vi "XML_EEG_writeHeader.vi"(8 "error in (no error)":errorcluster, 10 "XML_Header":T1, 11 "XML_EEG_File in":refnum<class "XML_EEG_File.lvclass">) -> (0 "error out":errorcluster, 2 "DOM document out":refnum<k20>, 3 "XML_EEG_File out":refnum<class "XML_EEG_File.lvclass">)   [LabVIEW 2016, in "XML_EEG_File_Parser.lvlib" / "XML_EEG_File.lvclass"]
uses:
  XML_EEG_File.lvclass
  XML_EEG_Header.ctl
  XML_EEG_File.lvclass/XML_EEG_File.ctl
  <vilib>/xml/NI_XML.lvlib
  <resource>/objmgr/DOMUserDefRef.rc
  XML_EEG_File_Parser.lvlib
panel:
  # "This VI is a part of BCI Design library, http://www.ru-bci.org \nCopyright © 2020, Sotnikov Peter, All rights reserved. License: CC BY-NC 4.0"
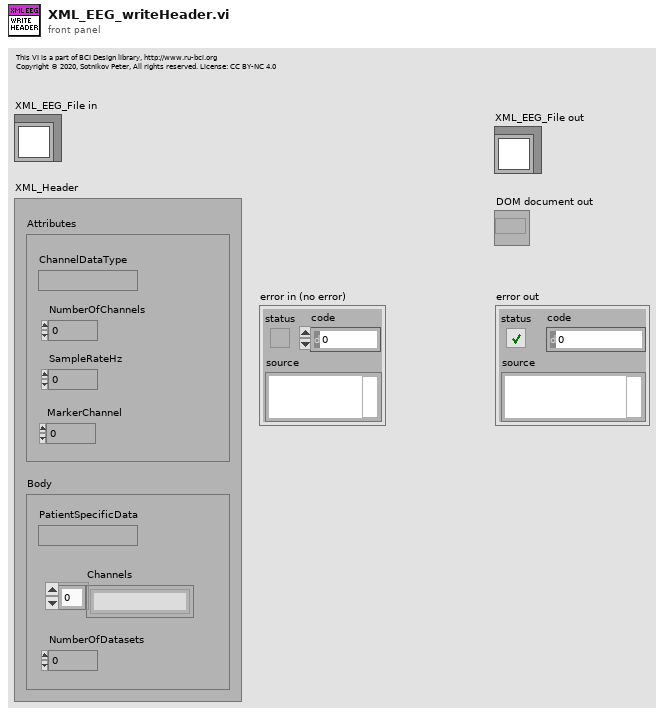
[diagram p1: front panel]
types:
  T1 = typedef "XML_EEG_File_Parser.lvlib/XML_EEG_Header.ctl" = cluster{"Attributes":cluster{"ChannelDataType":string, "NumberOfChannels":i32, "SampleRateHz":dbl, "MarkerChannel":i32}, "Body":cluster{"PatientSpecificData":string, "NumberOfDatasets":i32, "Channels":string[]}}
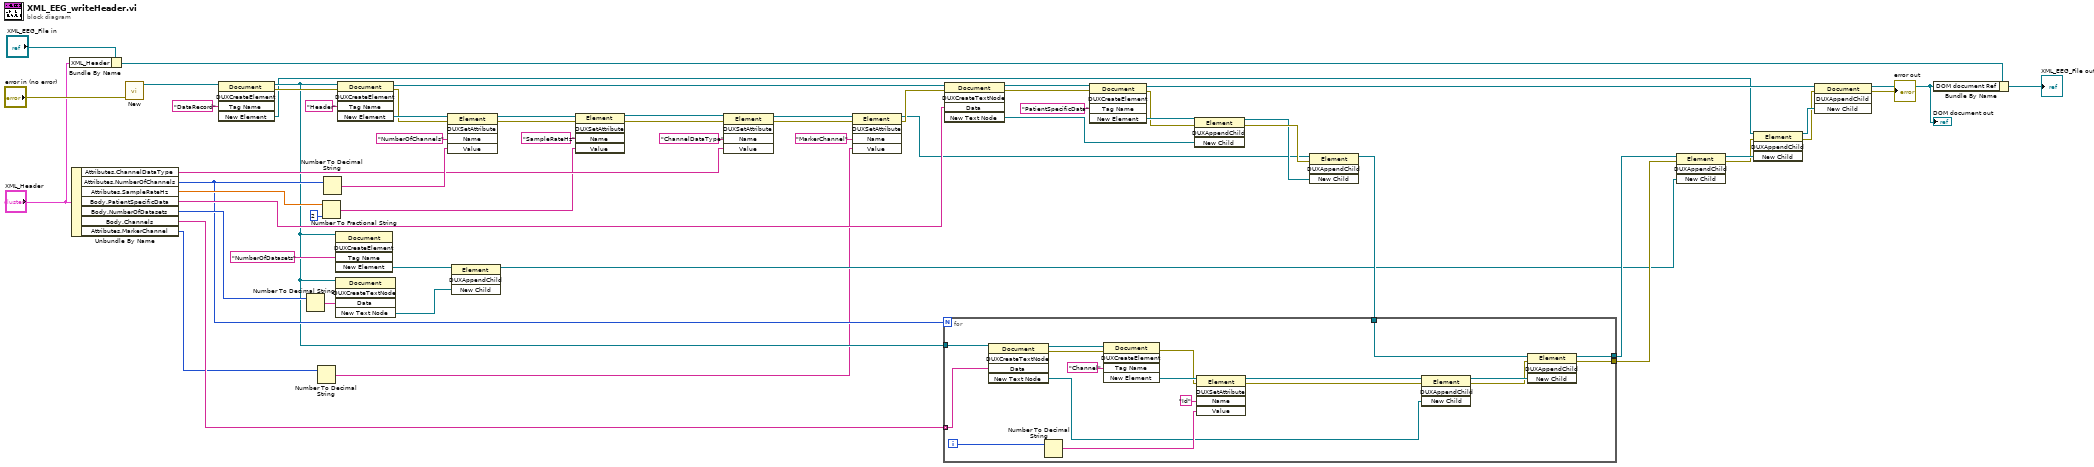
[diagram p0: block diagram]
diagram:
  n1 = Bundle By Name(cluster="XML_EEG_File in", "XML_Header"="XML_Header") -> (w3:refnum<class "XML_EEG_File.lvclass">)
  n2 = Unbundle By Name("XML_Header") -> ("Attributes.ChannelDataType"=w46:string, "Attributes.NumberOfChannels"=w26:i32, "Attributes.SampleRateHz"=w45:dbl, "Body.PatientSpecificData"=w41:string, "Body.NumberOfDatasets"=w30:i32, "Body.Channels"=w27:string[], "Attributes.MarkerChannel"=w8:i32)
  n3 = call <vilib>:"New.vi"("error in (no error)"="error in (no error)") -> ("DOM document out"=w60:refnum<k20>)  [unwired: 7 in, 1 out]
  n4 = invoke class="Document" method="DUXCreateElement"(reference=w60, "Tag Name"="DataRecord") -> (reference out=w25:refnum<k20>, error out=w58:errorcluster, "New Element"=w17:refnum<k20>)  [unwired: 3 in, 2 out]
  n5 = Number To Decimal String(number=w30) -> (decimal integer string=w31:string)  [unwired: 1 in]
  n6 = Number To Decimal String(number=w8) -> (decimal integer string=w7:string)  [unwired: 1 in]
  n7 = Number To Fractional String(number=w45, precision (6)=i16 2) -> (F-format string=w43:string)  [unwired: 2 in]
  n8 = Number To Decimal String(number=w26) -> (decimal integer string=w47:string)  [unwired: 1 in]
  n9 = invoke class="Document" method="DUXCreateElement"(reference=w25, "Tag Name"="NumberOfDatasets") -> ("New Element"=w29:refnum<k20>)  [unwired: 3 in, 4 out]
  n10 = invoke class="Document" method="DUXCreateTextNode"(reference=w25, "Data"=w31) -> ("New Text Node"=w28:refnum<k20>)  [unwired: 3 in, 4 out]
  n11 = invoke class="Document" method="DUXCreateElement"(reference=w25, error in=w58, "Tag Name"="Header") -> (reference out=w42:refnum<k20>, error out=w54:errorcluster, "New Element"=w56:refnum<k20>)  [unwired: 2 in, 2 out]
  n12 = invoke class="Element" method="DUXSetAttribute"(reference=w56, error in=w54, "Name"="NumberOfChannels", "Value"=w47) -> (reference out=w53:refnum<k20>, error out=w52:errorcluster)  [unwired: 1 in, 3 out]
  n13 = invoke class="Element" method="DUXAppendChild"(reference=w29, "New Child"=w28) -> (reference out=w21:refnum<k20>)  [unwired: 2 in, 3 out]
  n14 = invoke class="Element" method="DUXSetAttribute"(reference=w53, error in=w52, "Name"="SampleRateHz", "Value"=w43) -> (reference out=w50:refnum<k20>, error out=w49:errorcluster)  [unwired: 1 in, 3 out]
  n15 = invoke class="Element" method="DUXSetAttribute"(reference=w50, error in=w49, "Name"="ChannelDataType", "Value"=w46) -> (reference out=w11:refnum<k20>, error out=w12:errorcluster)  [unwired: 1 in, 3 out]
  n16 = invoke class="Element" method="DUXSetAttribute"(reference=w11, error in=w12, "Name"="MarkerChannel", "Value"=w7) -> (reference out=w9:refnum<k20>, error out=w10:errorcluster)  [unwired: 1 in, 3 out]
  n17 = invoke class="Document" method="DUXCreateTextNode"(reference=w42, error in=w10, "Data"=w41) -> (reference out=w39:refnum<k20>, error out=w40:errorcluster, "New Text Node"=w35:refnum<k20>)  [unwired: 2 in, 2 out]
  n18 = invoke class="Document" method="DUXCreateElement"(reference=w39, error in=w40, "Tag Name"="PatientSpecificData") -> (reference out=w20:refnum<k20>, error out=w36:errorcluster, "New Element"=w37:refnum<k20>)  [unwired: 2 in, 2 out]
  n19 = invoke class="Element" method="DUXAppendChild"(reference=w37, error in=w36, "New Child"=w35) -> (reference out=w33:refnum<k20>, error out=w34:errorcluster)  [unwired: 1 in, 2 out]
  n20 = invoke class="Element" method="DUXAppendChild"(reference=w9, error in=w34, "New Child"=w33) -> (reference out=w24:refnum<k20>)  [unwired: 1 in, 3 out]
  n21 = for {
    N: w26 -> [_]
    tunnel: w27 -> [w63] mode=indexing
    tunnel: w25 -> [w72]
    tunnel: w24 -> [w66]
    tunnel: [w65] -> w23
    tunnel: [w64] -> w22
    i -> [w74]
    n22 = invoke class="Document" method="DUXCreateTextNode"(reference=w72, "Data"=w63) -> (reference out=w71:refnum<k20>, error out=w70:errorcluster, "New Text Node"=w69:refnum<k20>)  [unwired: 3 in, 2 out]
    n23 = Number To Decimal String(number=w74) -> (decimal integer string=w73:string)  [unwired: 1 in]
    n24 = invoke class="Document" method="DUXCreateElement"(reference=w71, error in=w70, "Tag Name"="Channel") -> (error out=w76:errorcluster, "New Element"=w77:refnum<k20>)  [unwired: 2 in, 3 out]
    n25 = invoke class="Element" method="DUXSetAttribute"(reference=w77, error in=w76, "Name"="Id", "Value"=w73) -> (reference out=w61:refnum<k20>, error out=w62:errorcluster)  [unwired: 1 in, 3 out]
    n26 = invoke class="Element" method="DUXAppendChild"(reference=w61, error in=w62, "New Child"=w69) -> (reference out=w68:refnum<k20>, error out=w67:errorcluster)  [unwired: 1 in, 2 out]
    n27 = invoke class="Element" method="DUXAppendChild"(reference=w66, error in=w67, "New Child"=w68) -> (reference out=w64:refnum<k20>, error out=w65:errorcluster)  [unwired: 1 in, 2 out]
  }
  n28 = invoke class="Element" method="DUXAppendChild"(reference=w22, error in=w23, "New Child"=w21) -> (reference out=w19:refnum<k20>, error out=w18:errorcluster)  [unwired: 1 in, 2 out]
  n29 = invoke class="Element" method="DUXAppendChild"(reference=w17, error in=w18, "New Child"=w19) -> (reference out=w16:refnum<k20>, error out=w15:errorcluster)  [unwired: 1 in, 2 out]
  n30 = invoke class="Document" method="DUXAppendChild"(reference=w20, error in=w15, "New Child"=w16) -> (reference out=w1:refnum<k20>, error out=→"error out":errorcluster)  [unwired: 1 in, 2 out]
  "DOM document out" <- w1
  n31 = Bundle By Name(cluster=w3, "DOM document Ref"=w1) -> (→"XML_EEG_File out":refnum<class "XML_EEG_File.lvclass">)
